vi "FPGA Write IQ Data to FPGA.vi"(8 "error in (no error)":errorcluster, 11 "Sample Buffer":u8[](array[numeric])) -> (0 "error out":errorcluster)   [LabVIEW 2017]
doc: "This VI transfers the raw IIQ data samples to the FPGA for processing via a DMA FIFO"
uses:
  FPGA Global Variables.vi
  <vilib>/Utility/error.llb/Error Cluster From Error Code.vi
  <vilib>/rvi/errors/niLvFpgaAdjustHostInterfaceError.vi
  <vilib>/rvi/interface/nirviMethod/nirviMethod.xnode
  <vilib>/FPGAPlugInAG/Dynamic/niLvFpga_WriteFifo_Dynamic.vi
  <vilib>/rvi/errors/niLvFpgaMergeErrorWithErrorCode.vi
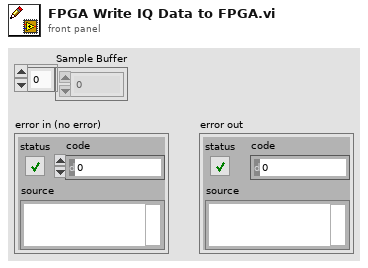
[diagram p1: front panel]
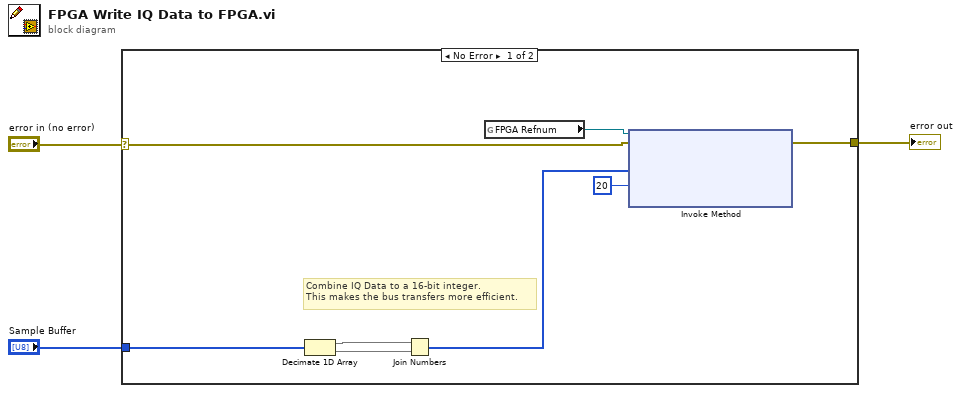
[diagram p0: block diagram]
diagram:
  n1 = case shown="No Error" "error in (no error)" {
    selector: "error in (no error)" -> [w10 w12]
    tunnel: [w11 w12] -> w1
    tunnel: "Sample Buffer" -> [w9 _]
    frame No Error {
      # "Combine IQ Data to a 16-bit integer.\nThis makes the bus transfers more efficient."
      n2 = Decimate 1D Array(w9) -> (w7:u8[], w8:u8[])
      n3 = Join Numbers(hi=w7, lo=w8) -> ((hi.lo)=w6:u16[])
      n4 = global read "FPGA Global Variables.vi" "FPGA Refnum"() -> (w5:refnum<k20>)
      n5 = xnode "Invoke Method"("FPGA VI Reference In"=w5, "error in"=w10, "Data"=w6, "Timeout (ms)"=20) -> ("error out"=w11:errorcluster)  [unwired: 2 out]
    }
    frame Error {
    }
  }
  "error out" <- w1
